vi "Set Field Ramp Rate.vi"(6 "Upper Bound (Model 430 only)":dbl=40.0, 7 "Segment (Model 430 only)":i32=1, 8 "error in":T2, 9 "Ramp Rate (kG/sec)":dbl format="%.3f", 11 "Communications Config":T1={"connection ID"=refnum, "IP"="192.168.0.108", "Active Comm Interface"=0, "Serial Port"="", "Programmer Type"=0, "connection ID"=refnum, "output cluster"={"GPIB address"=0, "GPIB bus"=0}} {"Programmer Type" items=["Model 430", "Model 420"]; "Active Comm Interface" items=["TCP/IP (Model 430 Only)", "RS232", "IEEE488"]}) -> (0 "error out":T2)   [LabVIEW 2017]
uses:
  commsControl.ctl
panel:
  out "output string":string
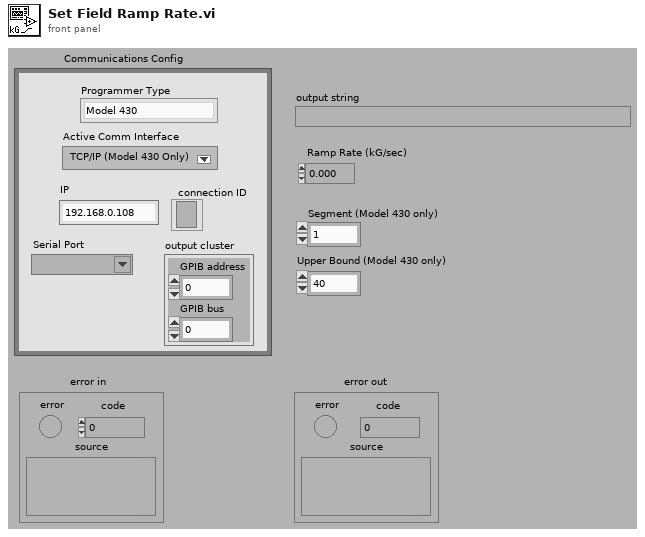
[diagram p1: front panel]
types:
  T1 = typedef "commsControl.ctl" = cluster{"connection ID":refnum<k5>, "IP":string, "Active Comm Interface":u16, "Serial Port":refnum<visa-resource-name>, "Programmer Type":u16, "connection ID":refnum<k5>, "output cluster":cluster{"GPIB address":i16, "GPIB bus":i16}}
  T2 = cluster{"error":bool, "code":i32, "source":string}
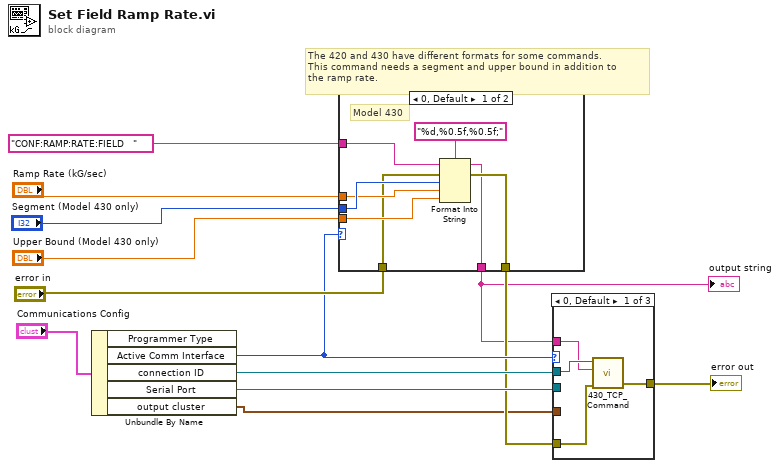
[diagram p0: block diagram]
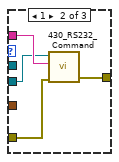
[diagram p2: hidden frame]
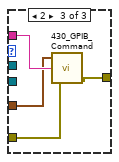
[diagram p3: hidden frame]
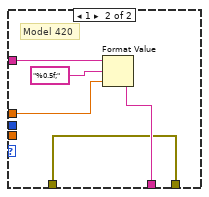
[diagram p4: hidden frame]
diagram:
  # "The 420 and 430 have different formats for some commands.\nThis command needs a segment and upper bound in addition to\nthe ramp rate."
  n1 = Unbundle By Name("Communications Config") -> ("Active Comm Interface"=w8:u16, "connection ID"=w6:refnum<k5>, "Serial Port"=w7:refnum<visa-resource-name>, "output cluster"=w1:cluster{"GPIB address":i16, "GPIB bus":i16})  [unwired: 1 out]
  n2 = case shown="0, Default" w8 {
    tunnel: "CONF:RAMP:RATE:FIELD   " -> [w18 w26]
    tunnel: "Ramp Rate (kG/sec)" -> [w20 w25]
    tunnel: [w15 w23] -> w4
    tunnel: "Upper Bound (Model 430 only)" -> [w19 _]
    tunnel: "Segment (Model 430 only)" -> [w21 _]
    tunnel: "error in" -> [w17 w22]
    tunnel: [w16 w22] -> w5
    frame 0, Default {
      # "Model 430"
      n3 = Format Into String(format string="%d,%0.5f,%0.5f;", initial string=w18, error in=w17, w21, w20, w19) -> (resulting string=w15:string, error out=w16:errorcluster)
    }
    frame 1 {
      # "Model 420"
      n4 = Format Value(string ("")=w26, format string="%0.5f;", value (0)=w25) -> (output string=w23:string)
    }
  }
  "output string" <- w4
  n5 = case shown="0, Default" w8 {
    tunnel: w4 -> [w29 w32 w38]
    tunnel: w5 -> [w28 w34 w37]
    tunnel: [w27 w33 w36] -> w3
    tunnel: w1 -> [_ _ w35]
    tunnel: w6 -> [w30 _ _]
    tunnel: w7 -> [_ w31 _]
    frame 0, Default {
      n6 = call "430_TCP_Command.vi"("error in (no error)"=w28, "Command"=w29, "connection ID"=w30) -> ("error out"=w27:errorcluster)  [unwired: 1 in, 2 out]
    }
    frame 1 {
      n7 = call "430_RS232_Command.vi"("error in (no error)"=w34, "Command"=w32, "VISA resource name"=w31) -> ("error out"=w33:errorcluster)  [unwired: 1 in, 2 out]
    }
    frame 2 {
      n8 = call "430_GPIB_Command.vi"("GPIB (In)"=w35, "Input command"=w38, "error in"=w37) -> ("error out"=w36:T2)  [unwired: 3 out]
    }
  }
  "error out" <- w3
